vi "Discrete Filter (DBL Array).vi"(2 "initialize":bool, 3 "filter coefficients":T1(array[cluster]) {"reverse coefficients" format="%.2f"; "forward coefficients" format="%.2f"}, 5 "input points":dbl[](array[numeric]) format="%.2f") -> (1 "output points":dbl[](array[numeric]) format="%.2f")   [LabVIEW 2020, in "NI_AdvCtrl_discrete linear.lvlib"]
doc: "LabVIEW no longer supports this VI. You can obtain similar functionality by installing the LabVIEW Simulation Module.\n\nFilters the set of input data using the direct form IIR filter specified by Reverse Coefficients and Forward Coefficients."
uses:
  <vilib>/addons/control/advanced/NI_AdvCtrl_discrete linear.lvlib
  <vilib>/addons/control/advanced/NI_AdvCtrl_continuous linear.lvlib
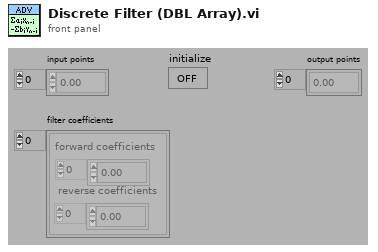
[diagram p1: front panel]
types:
  T1 = cluster{"forward coefficients":dbl[], "reverse coefficients":dbl[]}[]
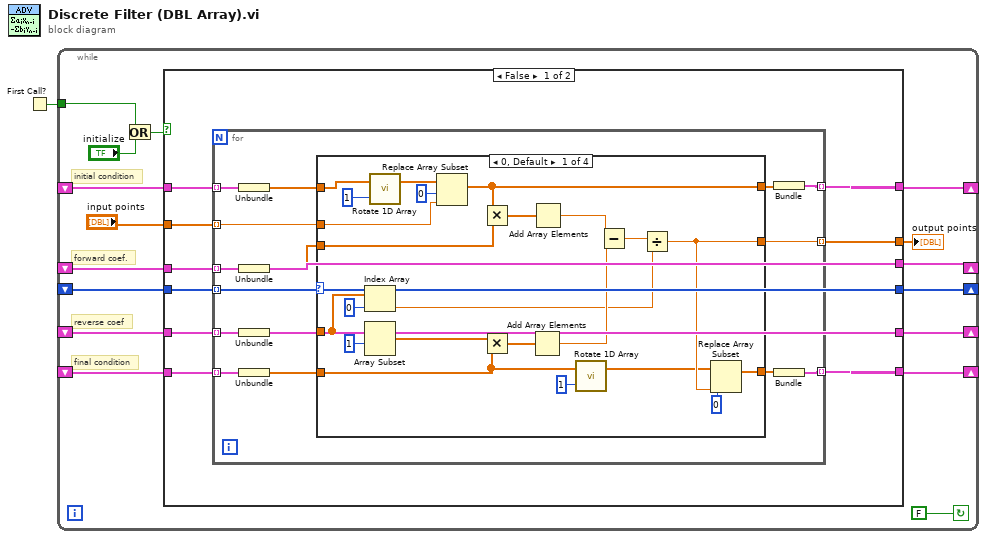
[diagram p0: block diagram]
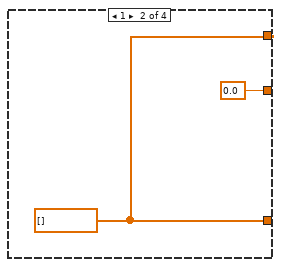
[diagram p2: hidden frame]
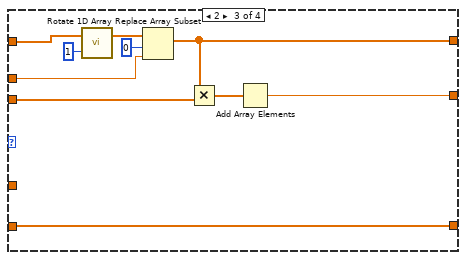
[diagram p3: hidden frame]
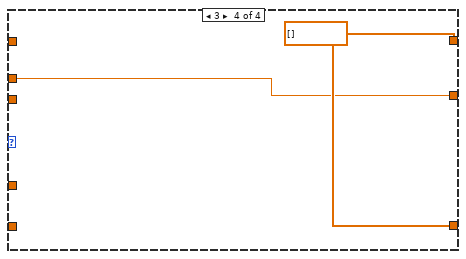
[diagram p4: hidden frame]
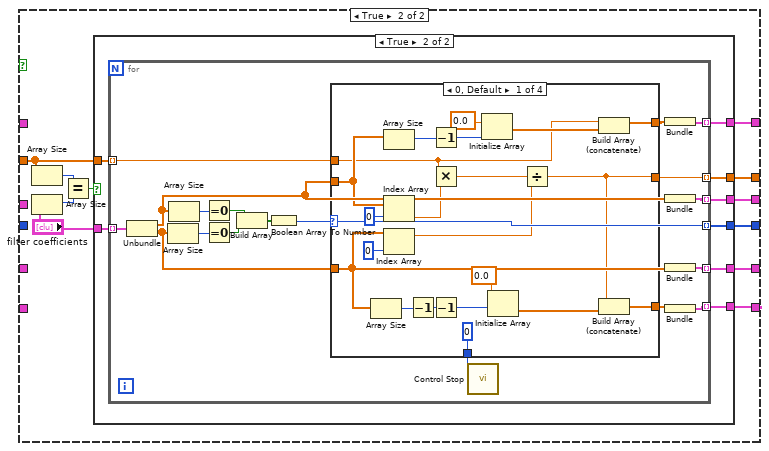
[diagram p5: hidden frame]
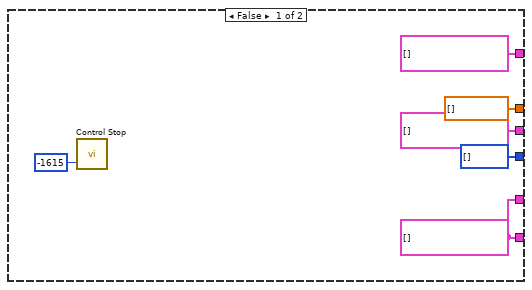
[diagram p6: hidden frame]
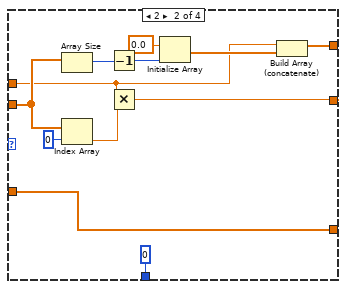
[diagram p7: hidden frame]
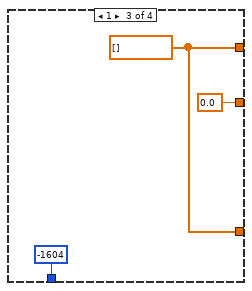
[diagram p8: hidden frame]
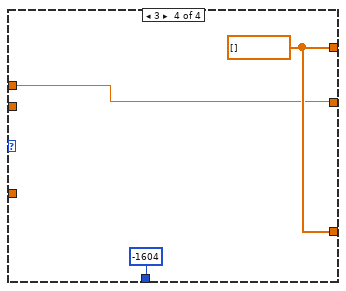
[diagram p9: hidden frame]
diagram:
  n1 = First Call?() -> (First Call?: T/F=w1:bool)
  n2 = while {
    shift-left: _ -> [w4]
    shift-right: [w5] -> _
    shift-left: _ -> [w7]
    shift-right: [w8] -> _
    shift-left: _ -> [w9]
    shift-right: [w10] -> _
    shift-left: _ -> [w12]
    shift-right: [w17] -> _
    shift-left: _ -> [w11]
    shift-right: [w16] -> _
    tunnel: w1 -> [w15]
    stop <- FALSE continue-if-true
    # "final condition"
    # "reverse coef"
    # "forward coef."
    # "initial condition"
    n3 = Or(x=w15, y="initialize") -> (x .or. y?=w13:bool)
    n4 = case shown="False" w13 {
      tunnel: w9 -> [w20 _]
      tunnel: w7 -> [w19 _]
      tunnel: w12 -> [w26 _]
      tunnel: w11 -> [w25 _]
      tunnel: [w21 w89] -> w3
      tunnel: [w24 w87] -> w17
      tunnel: [w23 w88] -> w16
      tunnel: "input points" -> [w22 w82]
      tunnel: [w20 w85] -> w10
      tunnel: [w19 w86] -> w8
      tunnel: [w18 w84] -> w5
      tunnel: w4 -> [w18 _]
      frame False {
        n5 = for {
          tunnel: w26 -> [w41] mode=indexing
          tunnel: w25 -> [w40] mode=indexing
          tunnel: [w32] -> w24 mode=indexing
          tunnel: [w28] -> w23 mode=indexing
          tunnel: w22 -> [w37] mode=indexing
          tunnel: [w36] -> w21 mode=indexing
          tunnel: w20 -> [w35] mode=indexing
          tunnel: w19 -> [w34] mode=indexing
          tunnel: w18 -> [w33] mode=indexing
          n6 = Unbundle(w41) -> ("array (last n elements first)"=w31:dbl[])
          n7 = Unbundle(w34) -> ("forward coefficients"=w30:dbl[])
          n8 = Unbundle(w35) -> ("reverse coefficients"=w29:dbl[])
          n9 = Unbundle(w40) -> ("reverse coefficients"=w27:dbl[])
          n10 = case shown="0, Default" w33 {
            tunnel: w31 -> [w46 _ w68 _]
            tunnel: w29 -> [w50 _ _ _]
            tunnel: w27 -> [w43 _ w70 _]
            tunnel: w30 -> [w56 _ w73 _]
            tunnel: [w57 w66 w71 w78] -> w39
            tunnel: [w59 w66 w70 w78] -> w38
            tunnel: w37 -> [w55 _ w74 w77]
            tunnel: [w52 0.0 ("Input_X") w72 w77] -> w36
            frame 0, Default {
              n11 = Index Array(array=w50, index=0 ("Index")) -> (element=w48:dbl)
              n12 = Array Subset(array=w50, index=1 ("Array Index")) -> (w54:dbl[])  [unwired: 1 in]
              n13 = call <vilib>:"Rotate 1D Array.vi"("n"=1, "array"=w46) -> ("array (last n elements first)"=w45:dbl[])  [unwired: 1 out]
              n14 = Replace Array Subset(array=w45, new element=w55, index=0 ("Index")) -> (w57:dbl[])
              n15 = Multiply(x=w57, y=w56) -> (x*y=w64:dbl[])
              n16 = Multiply(x=w54, y=w43) -> (x*y=w63:dbl[])
              n17 = Add Array Elements(numeric array=w63) -> (sum=w61:dbl)
              n18 = Add Array Elements(numeric array=w64) -> (sum=w62:dbl)
              n19 = call <vilib>:"Rotate 1D Array.vi"("n"=1, "array"=w43) -> ("array (last n elements first)"=w44:dbl[])  [unwired: 1 out]
              n20 = Subtract(x=w62, y=w61) -> (x-y=w51:dbl)
              n21 = Divide(x=w51, y=w48) -> (x/y=w52:dbl)
              n22 = Replace Array Subset(array=w44, new element=w52, index=0 ("Index")) -> (w59:dbl[])
            }
            frame 1 {
              w66 = dbl[] []
            }
            frame 2 {
              n23 = call <vilib>:"Rotate 1D Array.vi"("n"=1, "array"=w68) -> ("array (last n elements first)"=w69:dbl[])  [unwired: 1 out]
              n24 = Replace Array Subset(array=w69, new element=w74, index=0 ("Index")) -> (w71:dbl[])
              n25 = Multiply(x=w71, y=w73) -> (x*y=w76:dbl[])
              n26 = Add Array Elements(numeric array=w76) -> (sum=w72:dbl)
            }
            frame 3 {
              w78 = dbl[] []
            }
          }
          n27 = Bundle("array (last n elements first)"=w39) -> (w32:cluster{"array (last n elements first)":dbl[]})  [unwired: 1 in]
          n28 = Bundle("reverse coefficients"=w38) -> (w28:cluster{"reverse coefficients":dbl[]})  [unwired: 1 in]
        }
      }
      frame True {
        n29 = Array Size(array=w82) -> (size(s)=w81:i32)
        n30 = Array Size(array="filter coefficients") -> (size(s)=w80:i32)
        n31 = Equal?(x=w81, y=w80) -> (x = y?=w79:bool)
        n32 = case shown="True" w79 {
          tunnel: [dbl[] [] w103] -> w89
          tunnel: [w94 w102] -> w88
          tunnel: [cluster{dbl[]}[] [] w101] -> w87
          tunnel: w82 -> [_ w100]
          tunnel: [cluster{"Forward Coefficients":dbl[]}[] [] w99] -> w86
          tunnel: [w94 w98] -> w85
          tunnel: [u32[] [] w97] -> w84
          tunnel: "filter coefficients" -> [_ w96]
          frame False {
            w94 = cluster{"Reverse Coefficients":dbl[]}[] []
            n33 = call <vilib>:"Control Stop.vi"("error"=-1615) -> ()  [unwired: 2 out]
          }
          frame True {
            n34 = for {
              tunnel: [w121] -> w103 mode=indexing
              tunnel: [w107] -> w102 mode=indexing
              tunnel: [w109] -> w101 mode=indexing
              tunnel: w100 -> [w118] mode=indexing
              tunnel: [w108] -> w99 mode=indexing
              tunnel: [w106] -> w98 mode=indexing
              tunnel: [w110] -> w97 mode=indexing
              tunnel: w96 -> [w117] mode=indexing
              n35 = Unbundle(w117) -> ("forward coefficients"=w111:dbl[], "reverse coefficients"=w104:dbl[])
              n36 = Array Size(array=w104) -> (size(s)=w114:i32)
              n37 = Array Size(array=w111) -> (size(s)=w115:i32)
              n38 = Equal To 0?(x=w115) -> (x = 0?=w113:bool)
              n39 = Equal To 0?(x=w114) -> (x = 0?=w112:bool)
              n40 = Build Array(w113, w112) -> (w116:bool[])
              n41 = Boolean Array To Number(Boolean array=w116) -> (number=w110:u32)
              n42 = case shown="0, Default" w110 {
                tunnel: w111 -> [w134 w149 _ _]
                tunnel: [w127 w145 0.0 w159] -> w121
                tunnel: [w131 w146 w157 w160] -> w119
                tunnel: [w130 w143 w157 w160] -> w120
                tunnel: w118 -> [w132 w147 _ w159]
                tunnel: w104 -> [w122 w143 _ _]
                tunnel: [0 0 -1604 -1604] -> w105
                frame 0, Default {
                  n43 = Array Size(array=w122) -> (size(s)=w137:i32)
                  n44 = Array Size(array=w134) -> (size(s)=w142:i32)
                  n45 = Index Array(array=w134, index=0 ("Index")) -> (element=w138:dbl)
                  n46 = Index Array(array=w122, index=0 ("Index")) -> (element=w124:dbl)
                  n47 = Decrement(x=w137) -> (x-1=w128:i32)
                  n48 = Decrement(x=w142) -> (x-1=w141:i32)
                  n49 = Multiply(x=w132, y=w138) -> (x*y=w126:dbl)
                  n50 = Decrement(x=w128) -> (x-1=w136:i32)
                  n51 = Initialize Array(0.0 ("Element Data"), w141) -> (w133:dbl[])
                  n52 = Initialize Array(0.0 ("Element Data"), w136) -> (w129:dbl[])
                  n53 = Divide(x=w126, y=w124) -> (x/y=w127:dbl)
                  n54 = Build Array (concatenate)(w132, w133) -> (w131:dbl[])
                  n55 = Build Array (concatenate)(w127, w129) -> (w130:dbl[])
                }
                frame 2 {
                  n56 = Array Size(array=w149) -> (size(s)=w154:i32)
                  n57 = Index Array(array=w149, index=0 ("Index")) -> (element=w150:dbl)
                  n58 = Decrement(x=w154) -> (x-1=w153:i32)
                  n59 = Multiply(x=w147, y=w150) -> (x*y=w145:dbl)
                  n60 = Initialize Array(0.0 ("Element Data"), w153) -> (w148:dbl[])
                  n61 = Build Array (concatenate)(w147, w148) -> (w146:dbl[])
                }
                frame 1 {
                  w157 = dbl[] []
                }
                frame 3 {
                  w160 = dbl[] []
                }
              }
              n62 = call <vilib>:"Control Stop.vi"("error"=w105) -> ()  [unwired: 2 out]
              n63 = Bundle(w119) -> (w109:cluster{dbl[]})  [unwired: 1 in]
              n64 = Bundle("forward coefficients"=w111) -> (w108:cluster{"forward coefficients":dbl[]})  [unwired: 1 in]
              n65 = Bundle("reverse coefficients"=w104) -> (w106:cluster{"reverse coefficients":dbl[]})  [unwired: 1 in]
              n66 = Bundle("reverse coefficients"=w120) -> (w107:cluster{"reverse coefficients":dbl[]})  [unwired: 1 in]
            }
          }
        }
      }
    }
    "output points" <- w3
  }
